vi "Compare arrays for duplicates.vi"(7 "Tray count":i32=28, 8 "error in (no error)":errorcluster, 9 "Column (0-n)":i32, 10 "Add array":string[][](array[string]), 11 "Main array":string[][](array[string])) -> (0 "error out":errorcluster, 1 "add array dups?":bool, 2 "Dup Cnt":i32, 3 "Got duplicates?":bool)   [LabVIEW 2013]
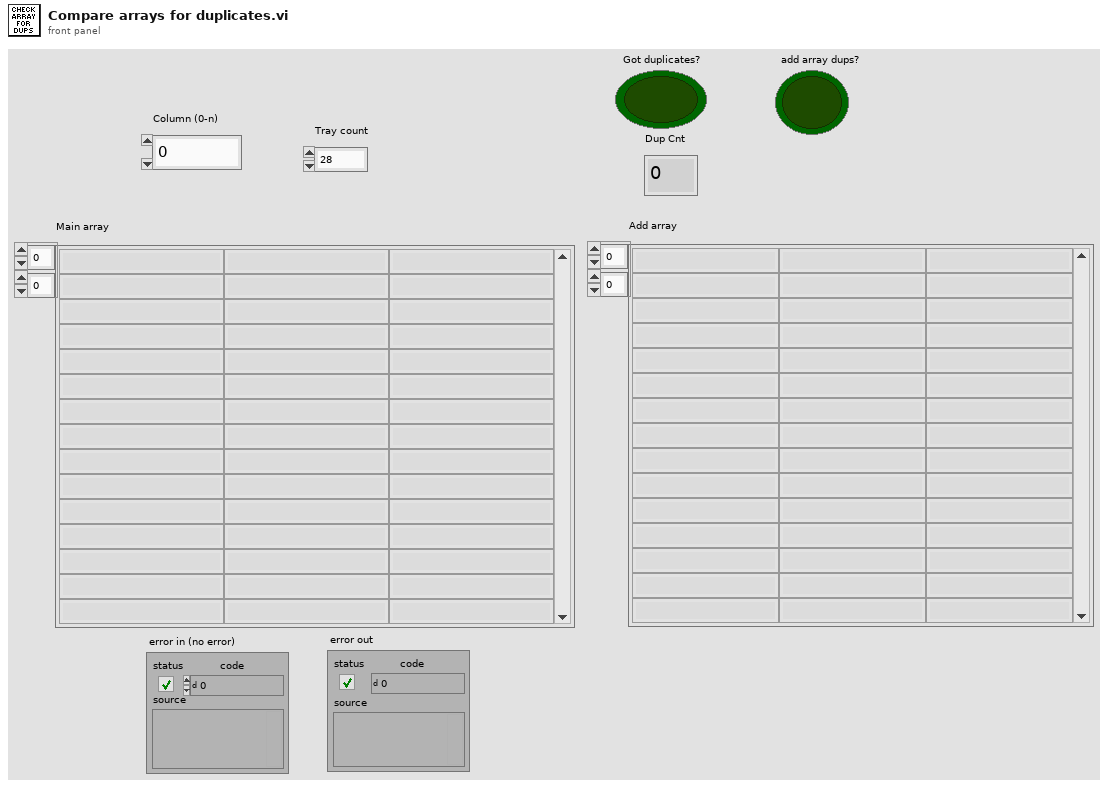
[diagram p1: front panel]
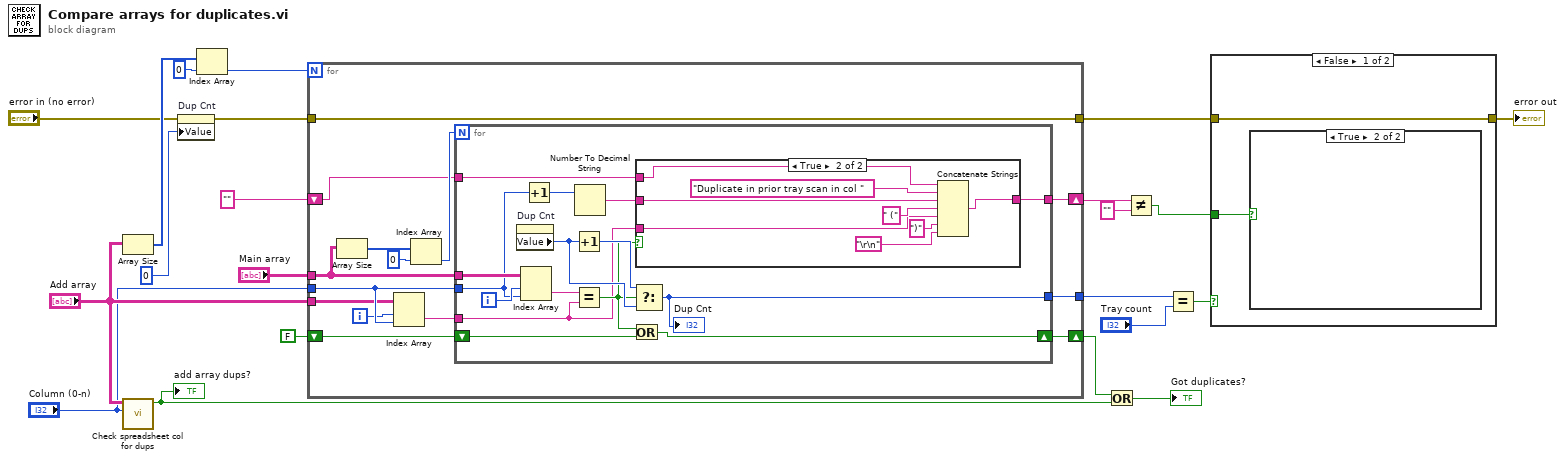
[diagram p0: block diagram]
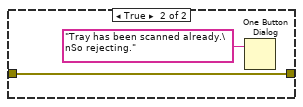
[diagram p3: hidden frame]
diagram:
  n1 = Array Size(array="Add array") -> (size(s)=w20:i32[])
  n2 = call "Check spreadsheet col for dups.vi"("col"="Column (0-n)", "Sorted Spreadsheet"="Add array") -> ("Got dups?"=w12:bool)  [unwired: 8 in, 1 out]
  "add array dups?" <- w12
  n3 = property on="Dup Cnt" class="DigNum (strict)"(error in="error in (no error)", "Value"=0 ("Dup Cnt")) -> (error out=w15:errorcluster)  [unwired: 1 in, 1 out]
  n4 = Index Array(array=w20, index=0) -> (element=w19:i32)
  n5 = for {
    N: w19 -> [_]
    tunnel: "Main array" -> [w33]
    tunnel: "Add array" -> [w30]
    tunnel: "Column (0-n)" -> [w32]
    shift-right: [w25] -> w5
    shift-left: FALSE -> [w28]
    tunnel: w15 -> [w27]
    tunnel: [w27] -> w6
    tunnel: [w26] -> w10
    shift-right: [w23] -> w3
    shift-left: "" -> [w24]
    i -> [w29]
    n6 = Array Size(array=w33) -> (size(s)=w36:i32[])
    n7 = Index Array(array=w30, index (row)=w29, index (col)=w32) -> (element=w31:string)
    n8 = Index Array(array=w36, index=0) -> (element=w34:i32)
    n9 = for {
      N: w34 -> [_]
      tunnel: w33 -> [w51]
      tunnel: w32 -> [w40]
      tunnel: w31 -> [w41]
      tunnel: [w45] -> w26
      shift-right: [w44] -> w25
      shift-left: w28 -> [w48]
      tunnel: w24 -> [w38]
      tunnel: [w37] -> w23
      i -> [w47]
      n10 = property on="Dup Cnt" class="DigNum (strict)"() -> ("Value"=w46:i32)  [unwired: 2 in, 2 out]
      n11 = Index Array(array=w51, index (row)=w47, index (col)=w40) -> (element=w50:string)
      n12 = Increment(x=w40) -> (x+1=w39:i32)
      n13 = Increment(x=w46) -> (x+1=w49:i32)
      n14 = Equal?(x=w50, y=w41) -> (x = y?=w43:bool)
      n15 = Number To Decimal String(number=w39) -> (decimal integer string=w42:string)  [unwired: 1 in]
      n16 = Or(x=w43, y=w48) -> (x .or. y?=w44:bool)
      n17 = Select(t=w49, s=w43, f=w46) -> (s? t:f=w45:i32)
      "Dup Cnt" <- w45
      n18 = case shown="True" w43 {
        tunnel: w42 -> [_ w59]
        tunnel: w41 -> [_ w57]
        tunnel: w38 -> [w52 w55]
        tunnel: [w52 w53] -> w37
        frame False {
        }
        frame True {
          n19 = Concatenate Strings(w55, "Duplicate in prior tray scan in col " ("string"), w59, " (" ("string"), w57, ")" ("string"), "\r\n") -> (w53:string)
        }
      }
    }
  }
  n20 = Or(x=w5, y=w12) -> (x .or. y?=→"Got duplicates?":bool)
  n21 = Not Equal?(x=w3, y="") -> (x != y?=w1:bool)
  n22 = Equal?(x=w10, y="Tray count") -> (x = y?=w8:bool)
  n23 = case shown="False" w8 {
    tunnel: [w62 w63] -> w7
    tunnel: w6 -> [w62 w63]
    tunnel: w1 -> [w61 _]
    frame False {
      n24 = case shown="True" w61 {
        frame False {
        }
        frame True {
        }
      }
    }
    frame True {
      n25 = One Button Dialog(message="Tray has been scanned already.\nSo rejecting.") -> ()  [unwired: 1 in, 1 out]
    }
  }
  "error out" <- w7
